vi "Error_to_Status_Cluster.vi"(1 "Error In":errorcluster, 2 "Status":T1) -> (0 "Status Cluster Out":T2)   [LabVIEW 2015]
uses:
  Status_Cluster.ctl
  Multi_Run_Status.ctl
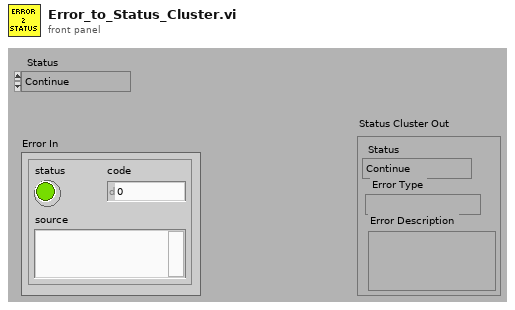
[diagram p1: front panel]
types:
  T1 = typedef "Multi_Run_Status.ctl" = enum16{"Continue", "Jump to Next Point", "Jump to Next Row", "Jump To Fall Back", "Terminate Run"}
  T2 = typedef "Status_Cluster.ctl" = cluster{"Status":T1, "Error Type":string, "Error Description":string}
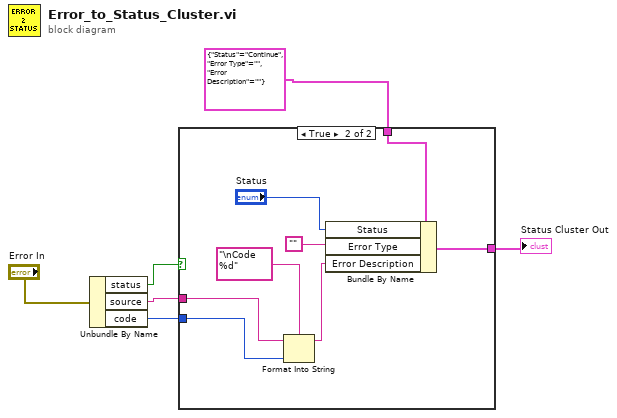
[diagram p0: block diagram]
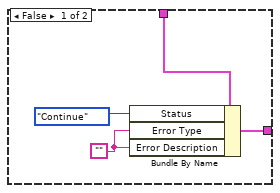
[diagram p2: hidden frame]
diagram:
  n1 = Unbundle By Name("Error In") -> ("status"=w4:bool, "source"=w2:string, "code"=w1:i32)
  n2 = case shown="True" w4 {
    tunnel: [w9 w17] -> w6
    tunnel: T2 {"Status"=enum."Continue", "Error Type"="", "Error Description"=""} ("Status Cluster Out") -> [w10 w18]
    tunnel: w2 -> [_ w13]
    tunnel: w1 -> [_ w14]
    frame False {
      w7 = ""
      n3 = Bundle By Name(cluster=w10, "Status"=Multi_Run_Status."Continue", "Error Type"=w7, "Error Description"=w7) -> (w9:T2)
    }
    frame True {
      n4 = Format Into String(format string="\nCode %d", initial string=w13, w14) -> (resulting string=w12:string)  [unwired: 1 in, 1 out]
      n5 = Bundle By Name(cluster=w18, "Status"="Status", "Error Type"="", "Error Description"=w12) -> (w17:T2)
    }
  }
  "Status Cluster Out" <- w6
